vi "Error.vi"(10 "error in (no error)":errorcluster, 11 "PQ Connection in":refnum<class "PQ Connection.lvclass">) -> (2 "error out":errorcluster, 3 "PQ Connection out":refnum<class "PQ Connection.lvclass">)   [LabVIEW 2013, in "PQ Connection.lvclass"]
uses:
  PQ Connection.lvclass
  PQ Connection.lvclass/PQ Connection.ctl
  libpq.dll
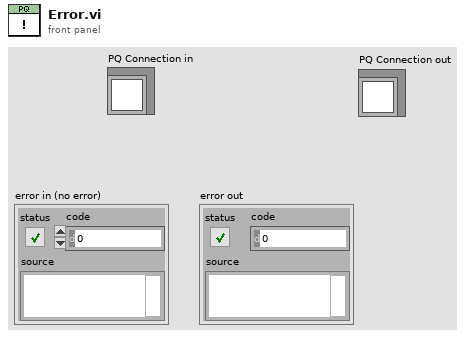
[diagram p1: front panel]
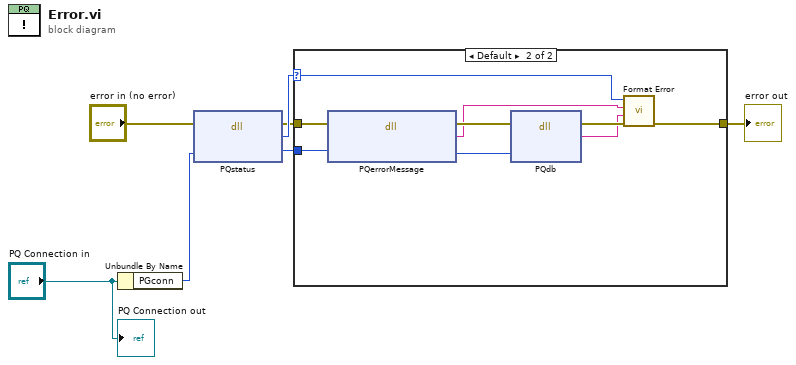
[diagram p0: block diagram]
diagram:
  n1 = Unbundle By Name("PQ Connection in") -> ("PGconn"=w6:u32)
  n2 = dll-call lib="C:/Users/patrick/Documents/GitHub/DSC/src/PostgreSQL Library/Connection/libpq.dll" fn="PQstatus"(error in="error in (no error)", "PGconn"=w6) -> (error out=w3:errorcluster, "PQstatus"=w5:u32, "PGconn"=w1:u32)  [unwired: 2 in, 1 out]
  n3 = case shown="Default" w5 {
    selector: w5 -> [_ w13]
    tunnel: w3 -> [w8 w17]
    tunnel: w1 -> [_ w16]
    tunnel: [w8 w11] -> w7
    frame 0 {
    }
    frame Default {
      n4 = dll-call lib="C:/Users/patrick/Documents/GitHub/DSC/src/PostgreSQL Library/Connection/libpq.dll" fn="PQerrorMessage"(error in=w17, "PGconn"=w16) -> (error out=w15:errorcluster, "Error Message"=w10:string, "PGconn"=w14:u32)  [unwired: 2 in, 1 out]
      n5 = dll-call lib="C:/Users/patrick/Documents/GitHub/DSC/src/PostgreSQL Library/Connection/libpq.dll" fn="PQdb"(error in=w15, "PGconn"=w14) -> (error out=w12:errorcluster, "Database"=w9:string)  [unwired: 3 in, 1 out]
      n6 = call "Format Error.vi"("error in (no error)"=w12, "Additional source description"=w9, "error message"=w10, "error code"=w13) -> ("error out"=w11:errorcluster)  [unwired: 7 in]
    }
  }
  "error out" <- w7
  "PQ Connection out" <- "PQ Connection in"
